vi "Populate Subpanels.vi"(8 "error in (no error)":errorcluster, 9 "View Labels (optional)":string[](array[string]), 10 "Views":refnum<class "Message Enqueuer.lvclass">[](array[class]), 11 "QuadViewManager In":refnum<class "QuadViewManager.lvclass">) -> (0 "error out":errorcluster, 3 "QuadViewManager Out":refnum<class "QuadViewManager.lvclass">)   [LabVIEW 2015, in "QuadViewManager.lvlib" / "QuadViewManager.lvclass"]
uses:
  QuadViewManager.lvclass
  <vilib>/ActorFramework/Message Enqueuer/Message Enqueuer.lvclass
  QuadViewManager.lvclass/QuadViewManager.ctl
  IViewable/IViewable Messages/Insert View Msg/Insert View Msg.lvclass/Insert View Msg.ctl
  <vilib>/ActorFramework/Message Enqueuer/Message Enqueuer.lvclass/Message Enqueuer.ctl
  <vilib>/ActorFramework/Message Enqueuer/Enqueue.vi
  <vilib>/ActorFramework/Message Priority Queue/Priority Enqueue.vi
  IViewManager/IViewManager/IViewManager.lvclass
  IViewable/IViewable Messages/Insert View Msg/Insert View Msg.lvclass
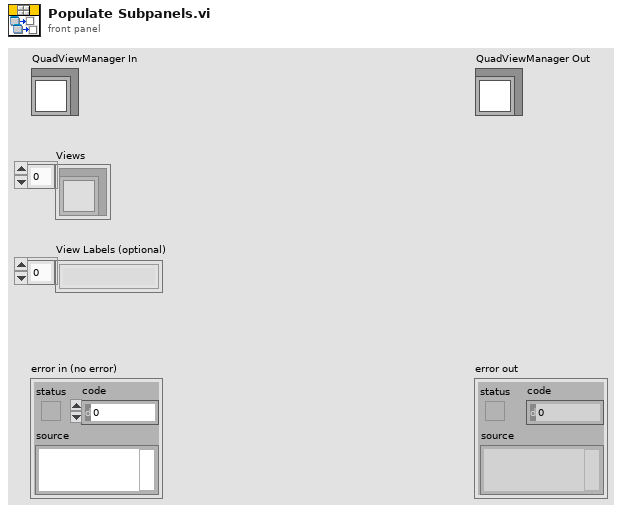
[diagram p1: front panel]
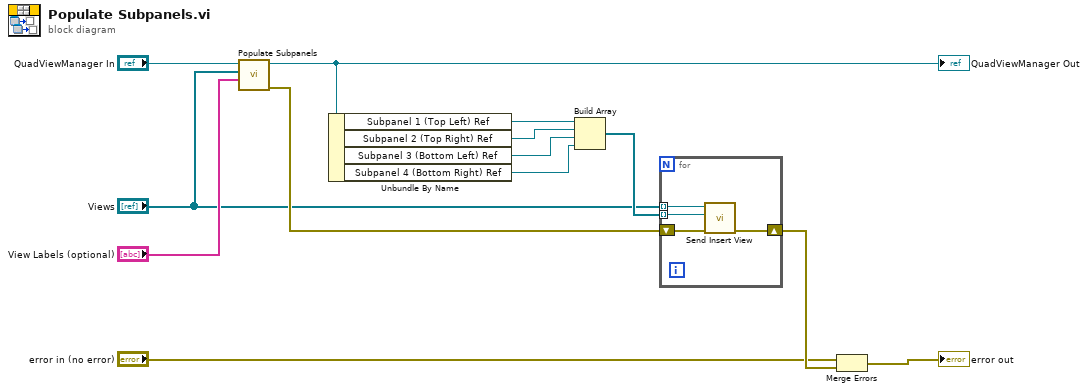
[diagram p0: block diagram]
diagram:
  n1 = call-parent "Populate Subpanels.vi"("View Labels (optional)"="View Labels (optional)", "Views"="Views", "IViewManager In"="QuadViewManager In") -> ("error out"=w3:errorcluster, "IViewManager Out"=w2:refnum<class "QuadViewManager.lvclass">)  [unwired: 7 in]
  "QuadViewManager Out" <- w2
  n2 = Unbundle By Name(w2) -> ("Subpanel 1 (Top Left) Ref"=w11:refnum<vi>, "Subpanel 2 (Top Right) Ref"=w8:refnum<vi>, "Subpanel 3 (Bottom Left) Ref"=w9:refnum<vi>, "Subpanel 4 (Bottom Right) Ref"=w10:refnum<vi>)
  n3 = Build Array(w11, w8, w9, w10) -> (w7:refnum<vi>[])
  n4 = for {
    tunnel: w7 -> [w17] mode=indexing
    shift-right: [w16] -> w6
    shift-left: w3 -> [w15]
    tunnel: "Views" -> [w14] mode=indexing
    n5 = call "Send Insert View.vi"("error in (no error)"=w15, "SubPnl Refnum"=w17, "Message Enqueuer"=w14) -> ("error out"=w16:errorcluster)  [unwired: 7 in, 1 out]
  }
  n6 = Merge Errors("error in (no error)", w6) -> (→"error out":errorcluster)
